vi "Read Linker Info.vi"(8 "error in (no error)":errorcluster, 11 "VI Path":path) -> (0 "error out":errorcluster, 3 "All VI Dependencies":string[](array[string]))   [LabVIEW 2019, in "Hawkeye.lvlib"]
uses:
  a9bd8d8a-b701-4855-97e4-326be6adfb7f.vi
  Hawkeye.lvlib
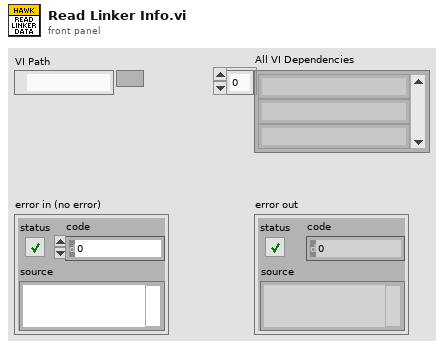
[diagram p1: front panel]
types:
  T1 = typedef "NI_FileType.lvlib/LVFileType.ctl" = enum32{"Invalid file", "Unknown type", "Instrument", "Control", "Polymorphic VI", "Project", "Library", "LVClass", "XControl", "XNode", "Shared library", ".NET assembly", "ActiveX interface", "CIN", "Run-time menu", "Palette menu", "Help file", "LLB", "XNode Edit Dependency", "Class Private Data Control", "Statechart", "MathScript .m file", "Ladder Diagram", "LVLibp", "XNode Build Dependency"}
  T2 = cluster{"path":path, "delimited name":string, "type":T1, "iState":u32, "iStyle":u16, "wStyle":u16, "buttons":u16, "viflags":u32, "viflags2":u32, "links":u32[]}[]
  T3 = cluster{"path":path, "delimited name":string, "type":T1, "iState":u32, "iStyle":u16, "wStyle":u16, "buttons":u16, "viflags":u32, "viflags2":u32, "links":u32[]}
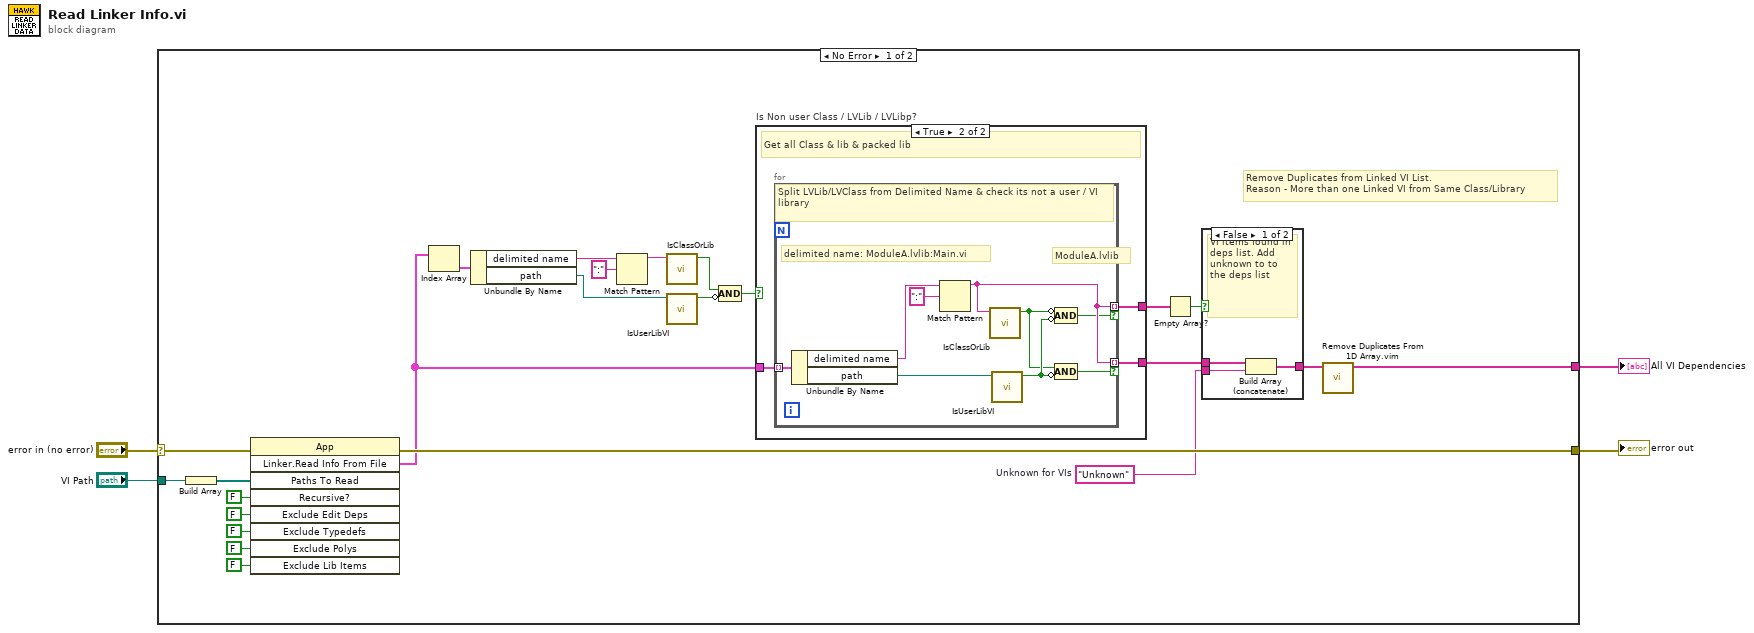
[diagram p0: block diagram]
diagram:
  n1 = case shown="No Error" "error in (no error)" {
    selector: "error in (no error)" -> [w17 w45]
    tunnel: "VI Path" -> [w18 _]
    tunnel: [w16 w45] -> w2
    tunnel: [w5 _] -> w1
    frame No Error {
      w7 = "Unknown"  # Unknown for VIs
      # "Remove Duplicates from Linked VI List.\nReason - More than one Linked VI from Same Class/Library"
      n2 = Build Array(w18) -> (w27:path[])
      n3 = invoke on="Invoke Node" class="App" method="Linker.Read Info From File"(error in=w17, "Paths To Read"=w27, "Recursive?"=FALSE, "Exclude Edit Deps"=FALSE ("Exclude Edit Time Dependencies"), "Exclude Typedefs"=FALSE, "Exclude Polys"=FALSE ("Exclude Poly VIs"), "Exclude Lib Items"=FALSE ("Exclude Unused Library Items")) -> (error out=w16:errorcluster, "Linker.Read Info From File"=w9:T2)  [unwired: 2 in, 7 out]
      n4 = Index Array(array=w9) -> (element=w8:T3)  [unwired: 1 in]
      n5 = Unbundle By Name(w8) -> ("delimited name"=w11:string, "path"=w13:path)
      n6 = Match Pattern(string=w11, regular expression=":") -> (before substring=w12:string)  [unwired: 1 in, 3 out]
      n7 = call "IsClassOrLib.vi"("LVFile Name"=w12) -> ("Is LVClass or Library?"=w14:bool)  [unwired: 9 in, 1 out]
      n8 = call "IsUserLibVI.vi"("ItemPath"=w13) -> ("IsUserLibVI?"=w15:bool)  [unwired: 10 in]
      n9 = Compound Arithmetic op=AND(w14, invert w15) -> (w6:bool)
      n10 = case "Is Non user Class / LVLib / LVLibp?" shown="True" w6 {
        tunnel: [_ w31] -> w26
        tunnel: [_ w30] -> w23
        tunnel: w9 -> [_ w29]
        frame False {
        }
        frame True {
          # "Get all Class & lib & packed lib"
          n11 = for {
            tunnel: w29 -> [w40] mode=indexing
            tunnel: [w37] -> w31 mode=indexing if=w35
            tunnel: [w37] -> w30 mode=indexing if=w34
            # "ModuleA.lvlib"
            # "delimited name: ModuleA.lvlib:Main.vi"
            # "Split LVLib/LVClass from Delimited Name & check its not a user / VI library"
            n12 = Unbundle By Name(w40) -> ("delimited name"=w38:string, "path"=w36:path)
            n13 = Match Pattern(string=w38, regular expression=":") -> (before substring=w37:string)  [unwired: 1 in, 3 out]
            n14 = call "IsClassOrLib.vi"("LVFile Name"=w37) -> ("Is LVClass or Library?"=w32:bool)  [unwired: 9 in, 1 out]
            n15 = call "IsUserLibVI.vi"("ItemPath"=w36) -> ("IsUserLibVI?"=w33:bool)  [unwired: 10 in]
            n16 = Compound Arithmetic op=AND(invert w32, invert w33) -> (w34:bool)
            n17 = Compound Arithmetic op=AND(w32, invert w33) -> (w35:bool)
          }
        }
      }
      n18 = Empty Array?(array=w23) -> (empty?=w25:bool)
      n19 = case shown="False" w25 {
        tunnel: w26 -> [w43 w44]
        tunnel: [w42 w44] -> w24
        tunnel: w7 -> [w41 _]
        frame False {
          # "VI items found in deps list. Add unknown to to the deps list"
          n20 = Build Array (concatenate)(w43, w41) -> (w42:string[])
        }
        frame True {
          # "Only class & lib in deps list"
        }
      }
      n21 = call "Remove Duplicates From 1D Array.vim"("array"=w24) -> ("array with duplicates removed"=w5:string[])  [unwired: 10 in]
    }
    frame Error {
    }
  }
  "error out" <- w2
  "All VI Dependencies" <- w1
